vi "test 9401 DIO Loop Back.vi"(8 "error in (no error)":errorcluster, 11 "TestCase in":refnum<class "Scan Engine EtherCAT System Tests.lvclass">) -> (0 "error out":errorcluster, 3 "TestCase out":refnum<class "Scan Engine EtherCAT System Tests.lvclass">)   [LabVIEW 2017, in "Scan Engine EtherCAT System Tests.lvclass"]
uses:
  Scan Engine EtherCAT System Tests.lvclass
  C:/Users/nitest/Desktop/Git/niveristand-custom-device-testing-tools/VeriStandTestCase/VeriStandTestCase.lvclass
  <vilib>/addons/_JKI Toolkits/VI Tester/TestCase.llb/TestCase.lvclass
  niveristand-custom-device-testing-tools/VeriStandTestCase/VeriStandTestCase.lvclass
  C:/Program Files (x86)/National Instruments/LabVIEW 2017/vi.lib/addons/_JKI Toolkits/VI Tester/TestCase.llb/TestCase.lvclass
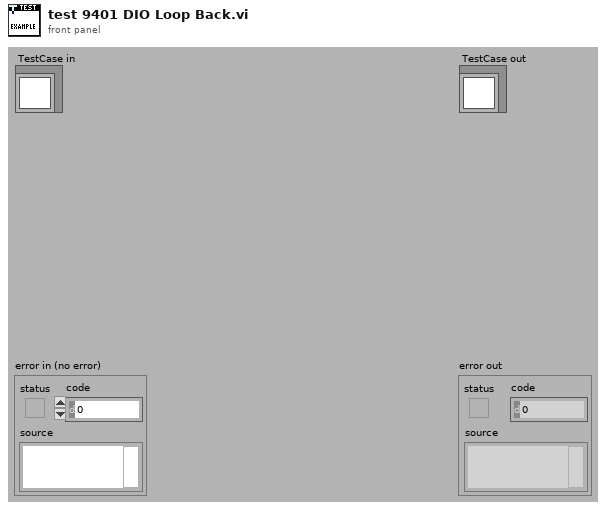
[diagram p1: front panel]
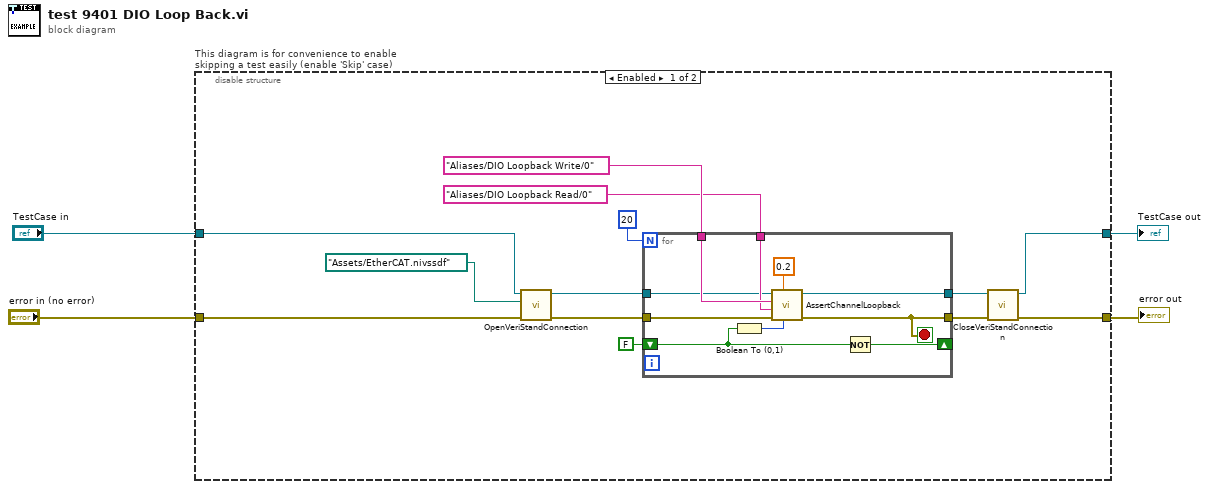
[diagram p0: block diagram]
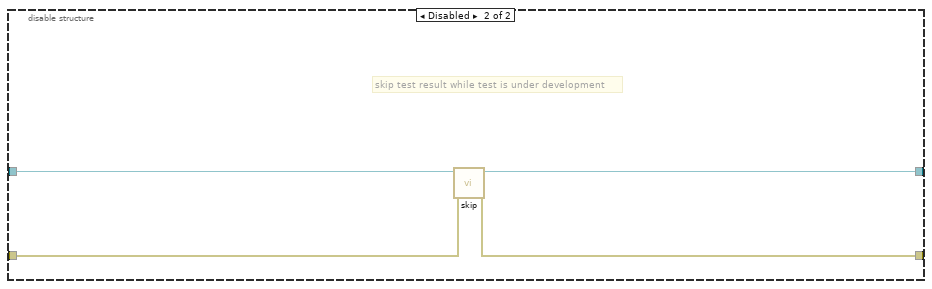
[diagram p2: hidden frame]
diagram:
  n1 = disable-structure "This diagram is for convenience to enable skipping a test easily (enable 'Skip' case)" shown="Enabled" {
    disable-tunnel: "TestCase in" -> [w9 w31]
    disable-tunnel: [w5 w29] -> w1
    disable-tunnel: [w6 w30] -> w3
    disable-tunnel: "error in (no error)" -> [w10 w28]
    frame Enabled {
      n2 = call-dynamic "OpenVeriStandConnection.vi"("error in (no error)"=w10, "System Definition File"=path "Assets/EtherCAT.nivssdf", "VeriStand Test Case in"=w9) -> ("error out"=w12:errorcluster, "VeriStand Test Case out"=w11:refnum<class "Scan Engine EtherCAT System Tests.lvclass">)  [unwired: 6 in, 1 out]
      n3 = for {
        N: 20 -> [_]
        tunnel: "Aliases/DIO Loopback Write/0" ("Channel") -> [w24]
        tunnel: [w22] -> w8
        tunnel: "Aliases/DIO Loopback Read/0" ("Channel") -> [w23]
        shift-right: [w27] -> _
        shift-left: FALSE -> [w26]
        tunnel: w12 -> [w25]
        tunnel: [w19] -> w7
        tunnel: w11 -> [w20]
        stop <- w22 stop-if-true
        n4 = Boolean To (0,1)(Boolean=w26) -> (0, 1=w21:i16)
        n5 = call "AssertChannelLoopback.vi"("Value"=w21, "Delay Time (s)"=0.2, "error in (no error)"=w25, "Read Channel"=w23, "Write Channel"=w24, "VeriStand Test Case in"=w20) -> ("error out"=w22:errorcluster, "VeriStand Test Case out"=w19:refnum<class "Scan Engine EtherCAT System Tests.lvclass">)  [unwired: 4 in]
        n6 = Not(x=w26) -> (.not. x?=w27:bool)
      }
      n7 = call-dynamic "CloseVeriStandConnection.vi"("error in (no error)"=w8, "VeriStand Test Case in"=w7) -> ("error out"=w6:errorcluster, "VeriStand Test Case out"=w5:refnum<class "Scan Engine EtherCAT System Tests.lvclass">)  [unwired: 8 in]
    }
    frame Disabled {
      # "skip test result while test is under development"
      n8 = call <vilib>:"skip.vi"("error in (no error)"=w28, "TestCase in"=w31) -> ("error out"=w30:errorcluster, "TestCase out"=w29:refnum<class "Scan Engine EtherCAT System Tests.lvclass">)  [unwired: 8 in]
    }
  }
  "error out" <- w3
  "TestCase out" <- w1
